vi "CoolPropTest.vi"(10 "HoejTryk":dbl=-1111111111.0 format="%#.6f", 11 "Lavtryk":dbl=-1111111111.0 format="%#.6f") -> (0 "log PH":T1, 1 "Punkt4":T2, 2 "Punkt3":T2, 3 "Punkt1":T2, 5 "Punkt2":T2)   [LabVIEW 2022 SP3]
uses:
  Coolprop_64bit/CoolProp_advanced.llb/FluidOfInterest.ctl
  Coolprop_64bit/Coolprop_lib.lvlib
  Coolprop_64bit/CoolProp_advanced.llb/FluidCommon.ctl
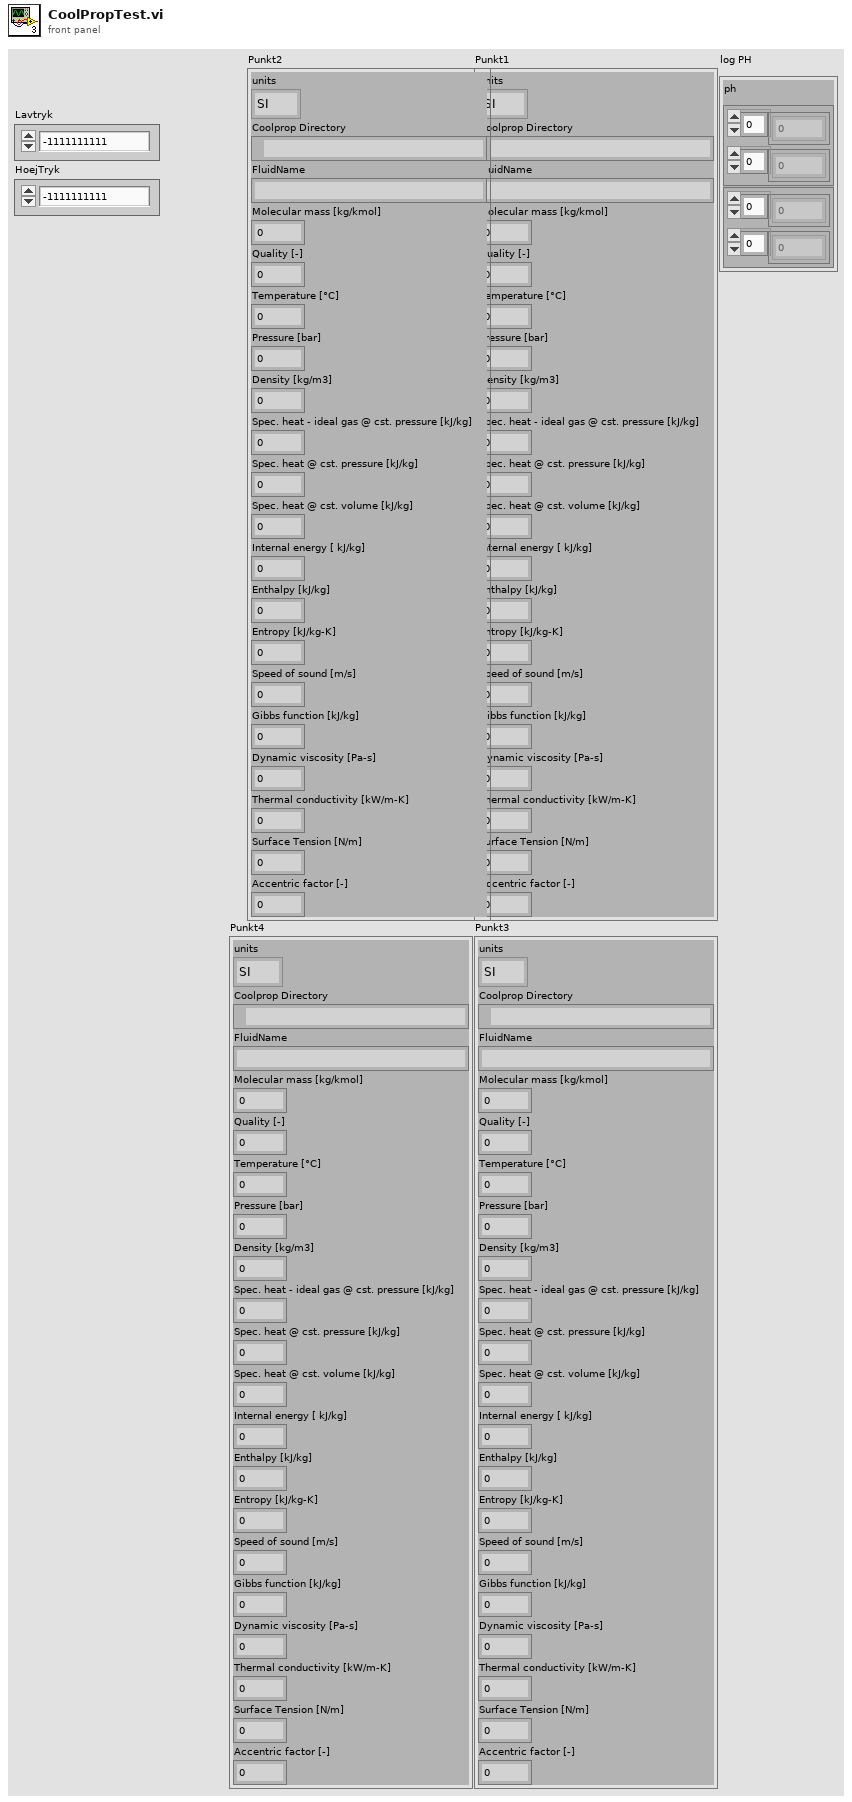
[diagram p1: front panel]
types:
  T1 = cluster{"ph":cluster{dbl[], dbl[]}, cluster{dbl[], dbl[]}}
  T2 = typedef "Coolprop_lib.lvlib/FluidCommon.ctl" = cluster{"units":enum16{"SI", "IP"}, "Coolprop Directory":path, "FluidName":string, "Molecular mass [kg/kmol]":dbl, "Quality [-]":dbl, "Temperature [°C]":dbl, "Pressure [bar]":dbl, "Density [kg/m3]":dbl, "Spec. heat - ideal gas @ cst. pressure [kJ/kg]":dbl, "Spec. heat @ cst. pressure [kJ/kg]":dbl, "Spec. heat @ cst. volume [kJ/kg]":dbl, "Internal energy [ kJ/kg]":dbl, "Enthalpy [kJ/kg]":dbl, "Entropy [kJ/kg-K]":dbl, "Speed of sound [m/s]":dbl, "Gibbs function [kJ/kg]":dbl, "Dynamic viscosity [Pa-s]":dbl, "Thermal conductivity [kW/m-K]":dbl, "Surface Tension [N/m]":dbl, "Accentric factor [-]":dbl}
  T3 = typedef "Coolprop_lib.lvlib/FluidOfInterest.ctl" = string
  T4 = enum16{"0", "TP", "TD", "PD", "TQ", "PQ", "HP", "SP", "SH"}
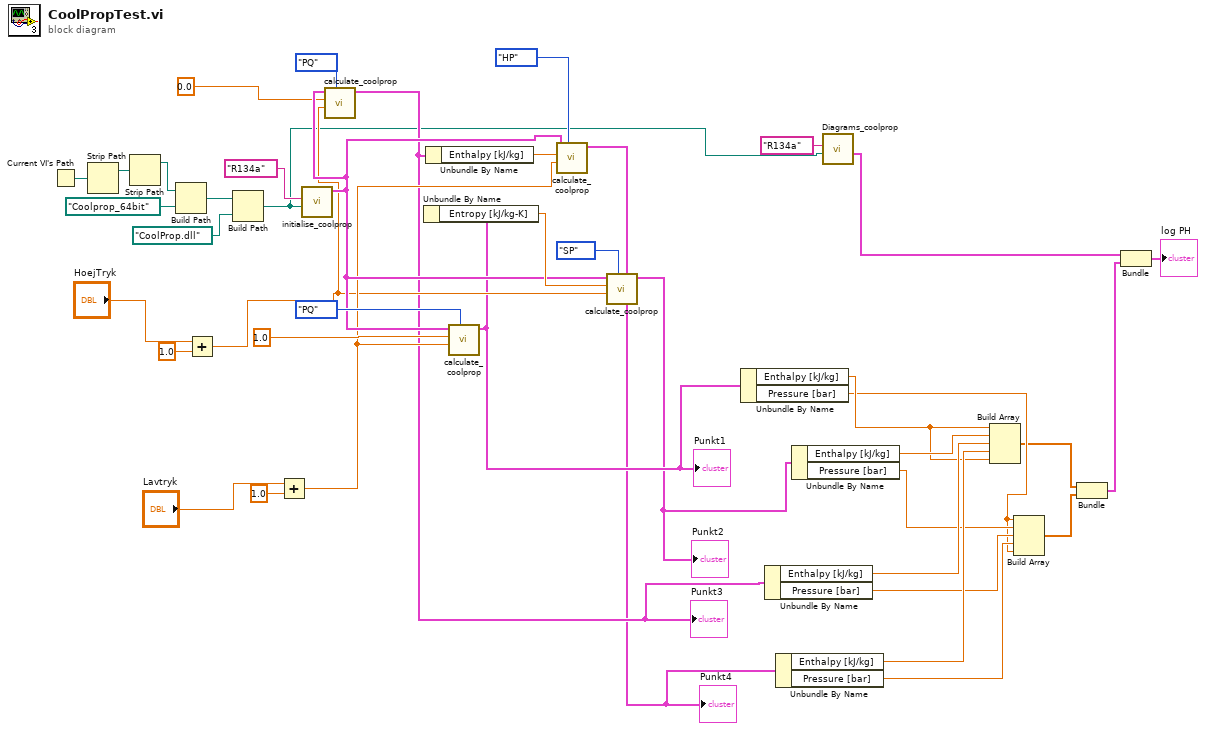
[diagram p0: block diagram]
diagram:
  n1 = Current VI's Path() -> (path=w40:path)
  n2 = Strip Path(path=w40) -> (stripped path=w39:path)  [unwired: 1 out]
  n3 = Strip Path(path=w39) -> (stripped path=w38:path)  [unwired: 1 out]
  n4 = Build Path(base path=w38, name or relative path=path "Coolprop_64bit") -> (appended path=w36:path)
  n5 = Add(x="HoejTryk", y=1.0) -> (x+y=w20:dbl)
  n6 = Build Path(base path=w36, name or relative path=path "CoolProp.dll") -> (appended path=w4:path)
  n7 = Add(x="Lavtryk", y=1.0) -> (x+y=w23:dbl)
  n8 = call "initialise_coolprop.vi"("Path to CoolProp.dll"=w4, "FluidOfInterest"=T3 "R134a") -> ("Common Out"=w28:T2)  [unwired: 7 in, 2 out]
  n9 = call "calculate_coolprop.vi"("InputCode"=T4."PQ", "Input_2"=w20, "Input_1"=0.0, "Common In"=w28) -> ("Common Out"=w17:T2)  [unwired: 3 in, 1 out]
  "Punkt3" <- w17
  n10 = Unbundle By Name(w17) -> ("Enthalpy [kJ/kg]"=w29:dbl)
  n11 = call "calculate_coolprop.vi"("InputCode"=T4."PQ", "Input_2"=w23, "Input_1"=1.0, "Common In"=w28) -> ("Common Out"=w19:T2)  [unwired: 3 in, 1 out]
  "Punkt1" <- w19
  n12 = Unbundle By Name(w19) -> ("Entropy [kJ/kg-K]"=w32:dbl)
  n13 = call "calculate_coolprop.vi"("InputCode"=T4."HP", "Input_2"=w23, "Input_1"=w29, "Common In"=w28) -> ("Common Out"=w16:T2)  [unwired: 3 in, 1 out]
  "Punkt4" <- w16
  n14 = call "calculate_coolprop.vi"("InputCode"=T4."SP", "Input_2"=w20, "Input_1"=w32, "Common In"=w28) -> ("Common Out"=w18:T2)  [unwired: 3 in, 1 out]
  "Punkt2" <- w18
  n15 = Unbundle By Name(w19) -> ("Enthalpy [kJ/kg]"=w12:dbl, "Pressure [bar]"=w8:dbl)
  n16 = Unbundle By Name(w17) -> ("Enthalpy [kJ/kg]"=w14:dbl, "Pressure [bar]"=w10:dbl)
  n17 = Unbundle By Name(w16) -> ("Enthalpy [kJ/kg]"=w13:dbl, "Pressure [bar]"=w9:dbl)
  n18 = Unbundle By Name(w18) -> ("Enthalpy [kJ/kg]"=w15:dbl, "Pressure [bar]"=w11:dbl)
  n19 = call "Diagrams_coolprop.vi"("Path"=w4, "FluidOfInterest"=T3 "R134a") -> ("ph"=w2:cluster{dbl[], dbl[]})  [unwired: 2 in, 7 out]
  n20 = Build Array(w12, w15, w14, w13, w12) -> (w7:dbl[])
  n21 = Build Array(w8, w11, w10, w9, w8) -> (w6:dbl[])
  n22 = Bundle(w7, w6) -> (w3:cluster{dbl[], dbl[]})  [unwired: 1 in]
  n23 = Bundle("ph"=w2, w3) -> (→"log PH":T1)  [unwired: 1 in]
